vi "tp3-2.vi"() -> ()   [LabVIEW 2013]
uses:
  <vilib>/sound2/lvsound2.llb/Sound Output Write (DBL).vi
panel:
  in  "Dial":dbl(knob)=150.0 scale=0.0..10000.0
  out "size(s)":i32
  out "Triangle":dbl[](graph)
  out "Rampa":dbl[](graph)
  out "Cuadrada":dbl[](graph)
  out "Senoidal":dbl[](graph)
  in  "Cluster":T1={"Sample rate (S/s)"=44100.0, "Number of channels"=2, "bits per sample"=16}
  in  "Stop Button":bool
  in  "Amplitud":dbl=1.0
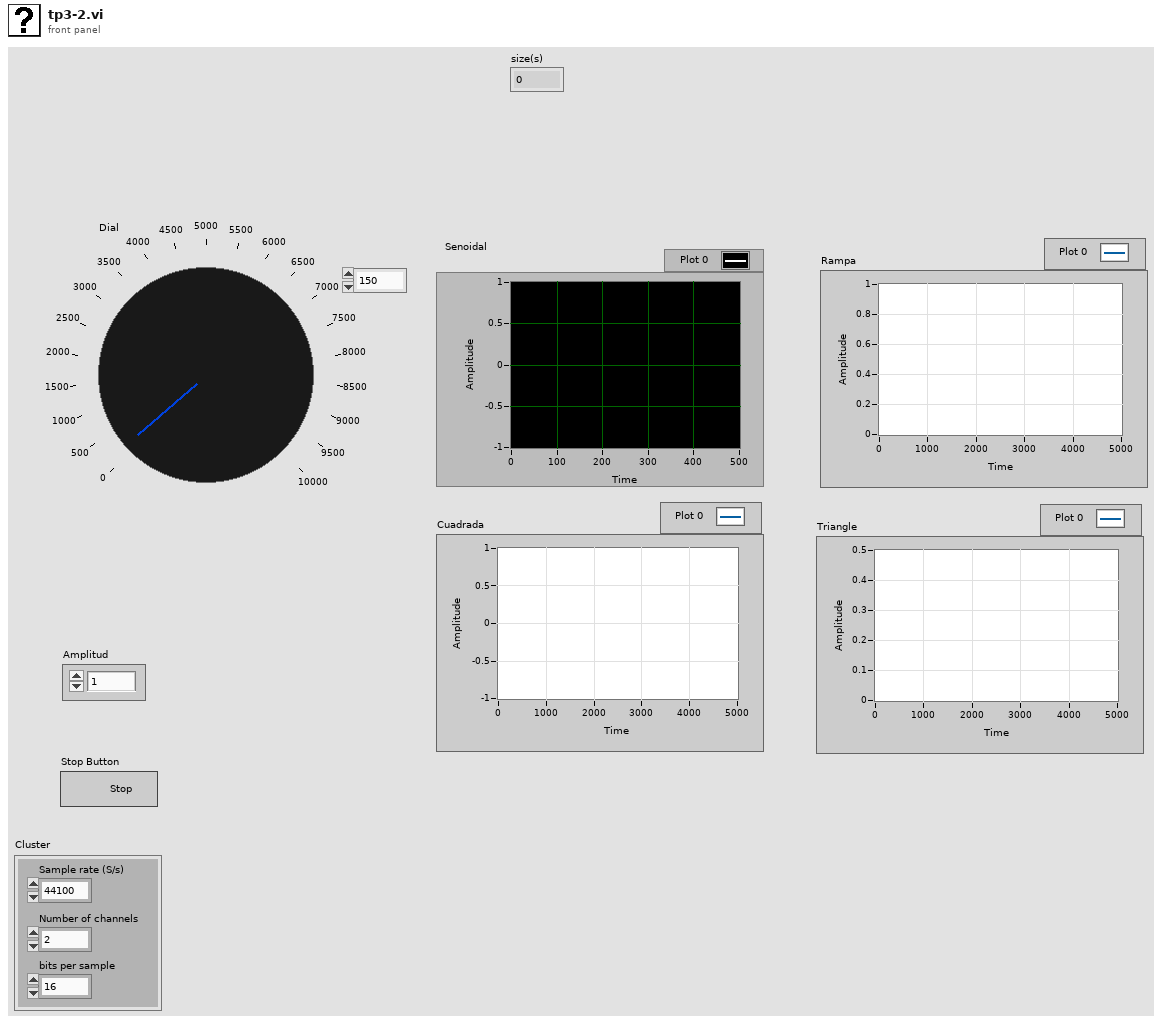
[diagram p1: front panel]
types:
  T1 = cluster{"Sample rate (S/s)":dbl, "Number of channels":i32, "bits per sample":i32}
  T2 = typedef "Sound Output Task ID.ctl" = u32
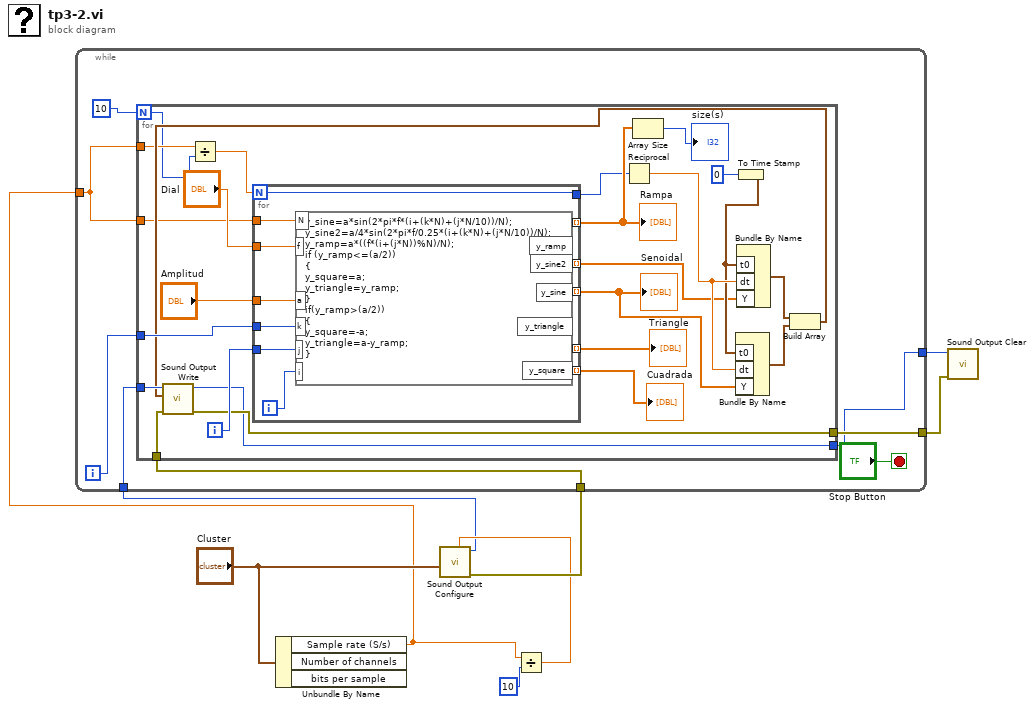
[diagram p0: block diagram]
diagram:
  n1 = Unbundle By Name("Cluster") -> ("Sample rate (S/s)"=w4:dbl)  [unwired: 2 out]
  n2 = Divide(x=w4, y=10) -> (x/y=w3:dbl)
  n3 = call <vilib>:"Sound Output Configure.vi"("number of samples/ch"=w3, "sound format"="Cluster") -> ("error out"=w6:errorcluster, "task ID"=w1:T2)  [unwired: 8 in]
  n4 = while {
    tunnel: w4 -> [w9]
    tunnel: w6 -> [w14]
    tunnel: [w11] -> w7
    tunnel: [w13] -> w2
    tunnel: w1 -> [w12]
    i -> [w15]
    stop <- "Stop Button" stop-if-true
    n5 = for {
      N: 10 -> [w20]
      tunnel: w15 -> [w40]
      tunnel: w14 -> [w38]
      tunnel: [w37] -> w13
      tunnel: w12 -> [w36]
      tunnel: [w35] -> w11
      tunnel: w9 -> [w21]
      tunnel: w9 -> [w17]
      i -> [w41]
      n6 = Divide(x=w21, y=w20) -> (x/y=w19:dbl)
      n7 = for {
        N: w19 -> [w45]
        tunnel: "Dial" -> [w53]
        tunnel: "Amplitud" -> [w52]
        tunnel: [w51] -> w26 mode=indexing
        tunnel: w41 -> [w49]
        tunnel: [w48] -> w28 mode=indexing
        tunnel: [w47] -> w24 mode=indexing
        tunnel: [w46] -> w27 mode=indexing
        tunnel: [w45] -> w22
        tunnel: [w44] -> w25 mode=indexing
        tunnel: w40 -> [w43]
        tunnel: w17 -> [w42]
        i -> [w50]
        n8 = formula code="y_sine=a*sin(2*pi*f*(i+(k*N)+(j*N/10))/N);\ny_sine2=a/4*sin(2*pi*f/0.25*(i+(k*N)+(j*N/10))/N);\ny_ramp=a*((f*(i+(j*N))%N)/N);\nif (y_ramp<=(a/2))\n{\ny_square=a;\ny_triangle=y_ramp;\n}\nif(y_ramp>(a/2))\n{\ny_square=-a;\ny_triangle=a-y_ramp;\n}"("f"=w53, "a"=w52, "N"=w42, "i"=w50, "j"=w49, "k"=w43) -> ("y_sine"=w51:dbl, "y_square"=w48:dbl, "y_ramp"=w47:dbl, "y_triangle"=w46:dbl, "y_sine2"=w44:dbl)
      }
      "Senoidal" <- w26
      "Cuadrada" <- w28
      "Rampa" <- w24
      "Triangle" <- w27
      n9 = Reciprocal(x=w22) -> (1/x=w33:dbl)
      n10 = Array Size(array=w24) -> (size(s)=→"size(s)":i32)
      n11 = To Time Stamp(1:0) -> (0:w32:timestamp)
      n12 = Bundle By Name("t0"=w32, "dt"=w33, "Y"=w26) -> (w31:waveform(dbl))  [unwired: 1 in]
      n13 = Bundle By Name("t0"=w32, "dt"=w33, "Y"=w25) -> (w30:waveform(dbl))  [unwired: 1 in]
      n14 = Build Array(w30, w31) -> (w23:waveform(dbl)[])
      n15 = call-poly <vilib>:"Sound Output Write.vi"("error in (no error)"=w38, "data"=w23, "task ID"=w36) -> ("error out"=w37:errorcluster, "task ID out"=w35:T2)  [unwired: 7 in]
    }
  }
  n16 = call <vilib>:"Sound Output Clear.vi"("error in (no error)"=w2, "task ID"=w7) -> ()  [unwired: 9 in, 1 out]
